vi "GetSpectrometerNameFromMP.vi"(1 "MP Pos":i32) -> (0 "String":string)   [LabVIEW 2018]
uses:
  Global Variables.vi
  <vilib>/Utility/file.llb/Read Delimited Spreadsheet (string).vi
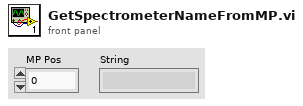
[diagram p1: front panel]
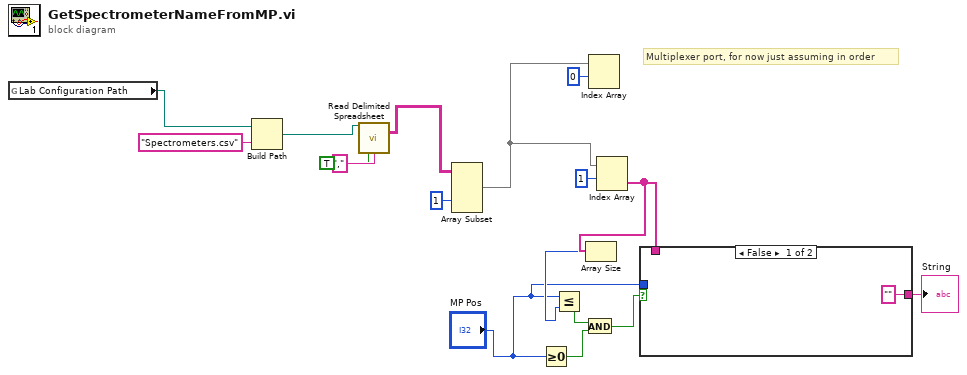
[diagram p0: block diagram]
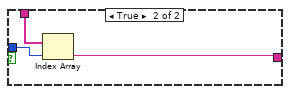
[diagram p2: hidden frame]
diagram:
  # "Multiplexer port, for now just assuming in order"
  n1 = global read "Global Variables.vi" "Lab Configuration Path"() -> (w17:path)
  n2 = Build Path(base path=w17, name or relative path="Spectrometers.csv") -> (appended path=w15:path)
  n3 = call-poly <vilib>:"Read Delimited Spreadsheet.vi"("file path (dialog if empty)"=w15, "transpose? (F)"=TRUE, "delimiter (\\t)"="," ("delimiter (\\t)")) -> ("all rows"=w12:string[][])  [unwired: 7 in, 5 out]
  n4 = Array Subset(array=w12, index (col)=1 ("index")) -> (w10:string[][])  [unwired: 3 in]
  n5 = Greater Or Equal To 0?(x="MP Pos") -> (x >= 0?=w4:bool)
  n6 = Index Array(array=w10, index (row)=0) -> ()  [unwired: 1 in, 1 out]
  n7 = Index Array(array=w10, index (row)=1) -> (element=w7:string[])  [unwired: 1 in]
  n8 = Array Size(array=w7) -> (size(s)=w6:i32)
  n9 = Less Or Equal?(x="MP Pos", y=w6) -> (x <= y?=w5:bool)
  n10 = And(x=w5, y=w4) -> (x .and. y?=w3:bool)
  n11 = case shown="False" w3 {
    tunnel: w7 -> [_ w21]
    tunnel: ["" ("String") w20] -> w2
    tunnel: "MP Pos" -> [_ w19]
    frame False {
    }
    frame True {
      n12 = Index Array(array=w21, index=w19) -> (element=w20:string)
    }
  }
  "String" <- w2
